vi "4-20mA.vi"(8 "error in (no error)":errorcluster, 10 "Reg array":u16[](array[numeric]), 11 "object in":refnum<class "Pressure-Transducer.lvclass">) -> (0 "error out":errorcluster, 1 "Array size":i32, 2 "4-20mA Array":dbl[](array[numeric]), 3 "object out":refnum<class "Pressure-Transducer.lvclass">)   [LabVIEW 2021, in "Pressure-Transducer.lvclass"]
uses:
  Pressure-Transducer.lvclass
panel:
  # "Conversion for 4 to 20mA transducer \nfor the adam 4017+\n\nOutput the 4mA been subtracted"
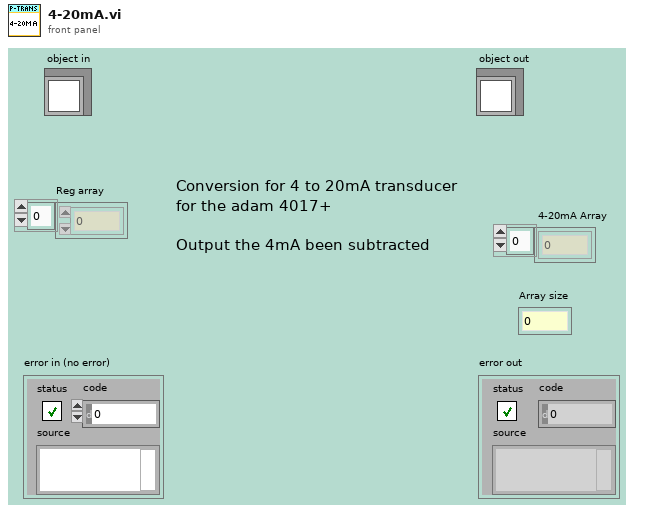
[diagram p1: front panel]
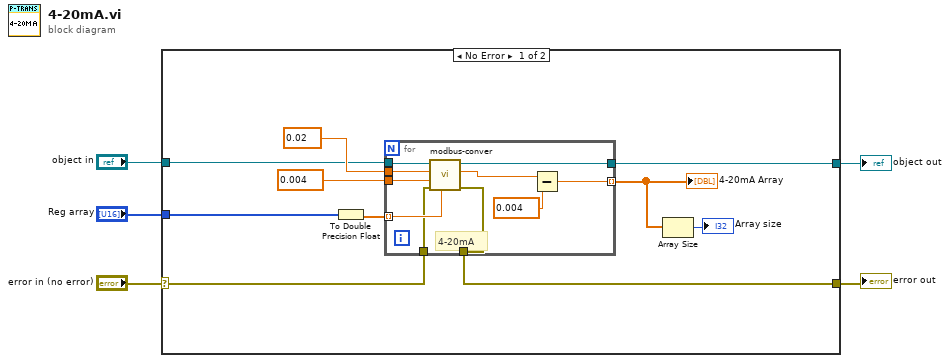
[diagram p0: block diagram]
diagram:
  n1 = case shown="No Error" "error in (no error)" {
    selector: "error in (no error)" -> [w10 w27]
    tunnel: [w9 w27] -> w4
    tunnel: [w11 w26] -> w2
    tunnel: "object in" -> [w12 w26]
    tunnel: "Reg array" -> [w8 _]
    frame No Error {
      n2 = To Double Precision Float(number=w8) -> (double precision float=w15:dbl[])
      n3 = for {
        tunnel: [w17] -> w7 mode=indexing
        tunnel: [w24] -> w11
        tunnel: w12 -> [w23]
        tunnel: 0.02 ("Scale Max Range") -> [w22]
        tunnel: 0.004 ("Scale Max Range") -> [w21]
        tunnel: w15 -> [w20] mode=indexing
        tunnel: w10 -> [w19]
        tunnel: [w18] -> w9
        # "4-20mA"
        n4 = call-dynamic "modbus-conver.vi"("Reg"=w20, "error in (no error)"=w19, "Scale Min range"=w21, "Scale Max Range"=w22, "object in"=w23) -> ("error out"=w18:errorcluster, "output"=w25:dbl, "object out"=w24:refnum<class "Pressure-Transducer.lvclass">)  [unwired: 4 in]
        n5 = Subtract(x=w25, y=0.004) -> (x-y=w17:dbl)
      }
      "4-20mA Array" <- w7
      n6 = Array Size(array=w7) -> (size(s)=→"Array size":i32)
    }
    frame Error {
    }
  }
  "error out" <- w4
  "object out" <- w2
